vi "Teste234.vi"() -> ()   [LabVIEW 2019]
panel:
  out "tubo":i32(slide) scale=0.0..1950.0
  out "String lida em Caracter":string
  in  "home":bool
  in  "123":bool
  out "Altura Momentânea":i32
  in  "Parar":bool
  in  "Iniciar":bool
  in  "MWU2987":i16
  in  "MWU2986":i16
  in  "MWU2985":i16
  in  "MWU2984":i16
  in  "MWU2983":i16
  in  "MWU2982":i16
  in  "MWU2981":i16
  in  "MWU2980":i16
  in  "MWU2979":i16
  in  "MWU2978":i16
  in  "MWU2977":i16
  in  "MWU2976":i16
  in  "MWU2975":i16
  out "MWU1100":i16
  # "TESTE 234"
  # "mm"
  # "Teste destinado para verificar \no funcionamento mínimo do \nsistema\n Ao apertar em Iniciar, o sensor \nirá subir até 234mm e ficará \naguardando o usuário apertar o \nbotão HOME"
  # "Comando enviado"
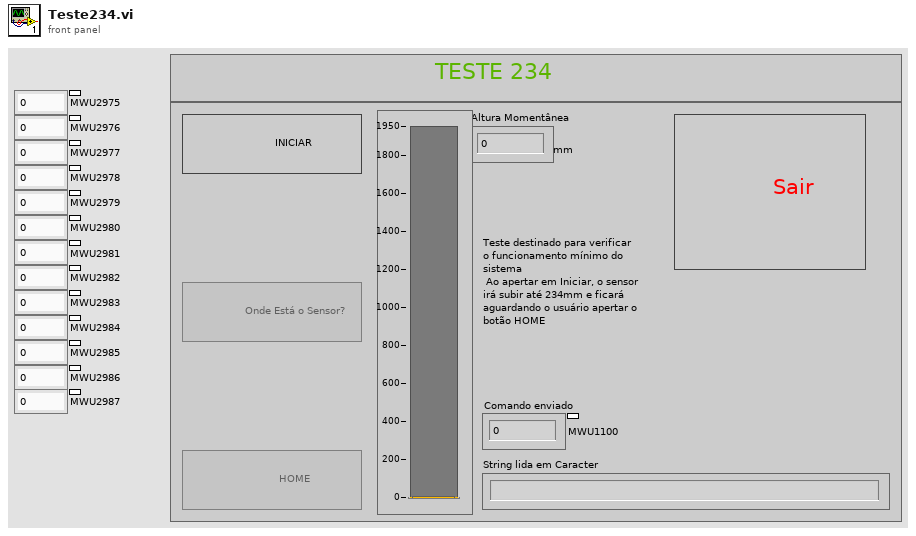
[diagram p1: front panel]
types:
  T1 = enum8{"Enabled", "Disabled", "Disabled and Grayed Out"}
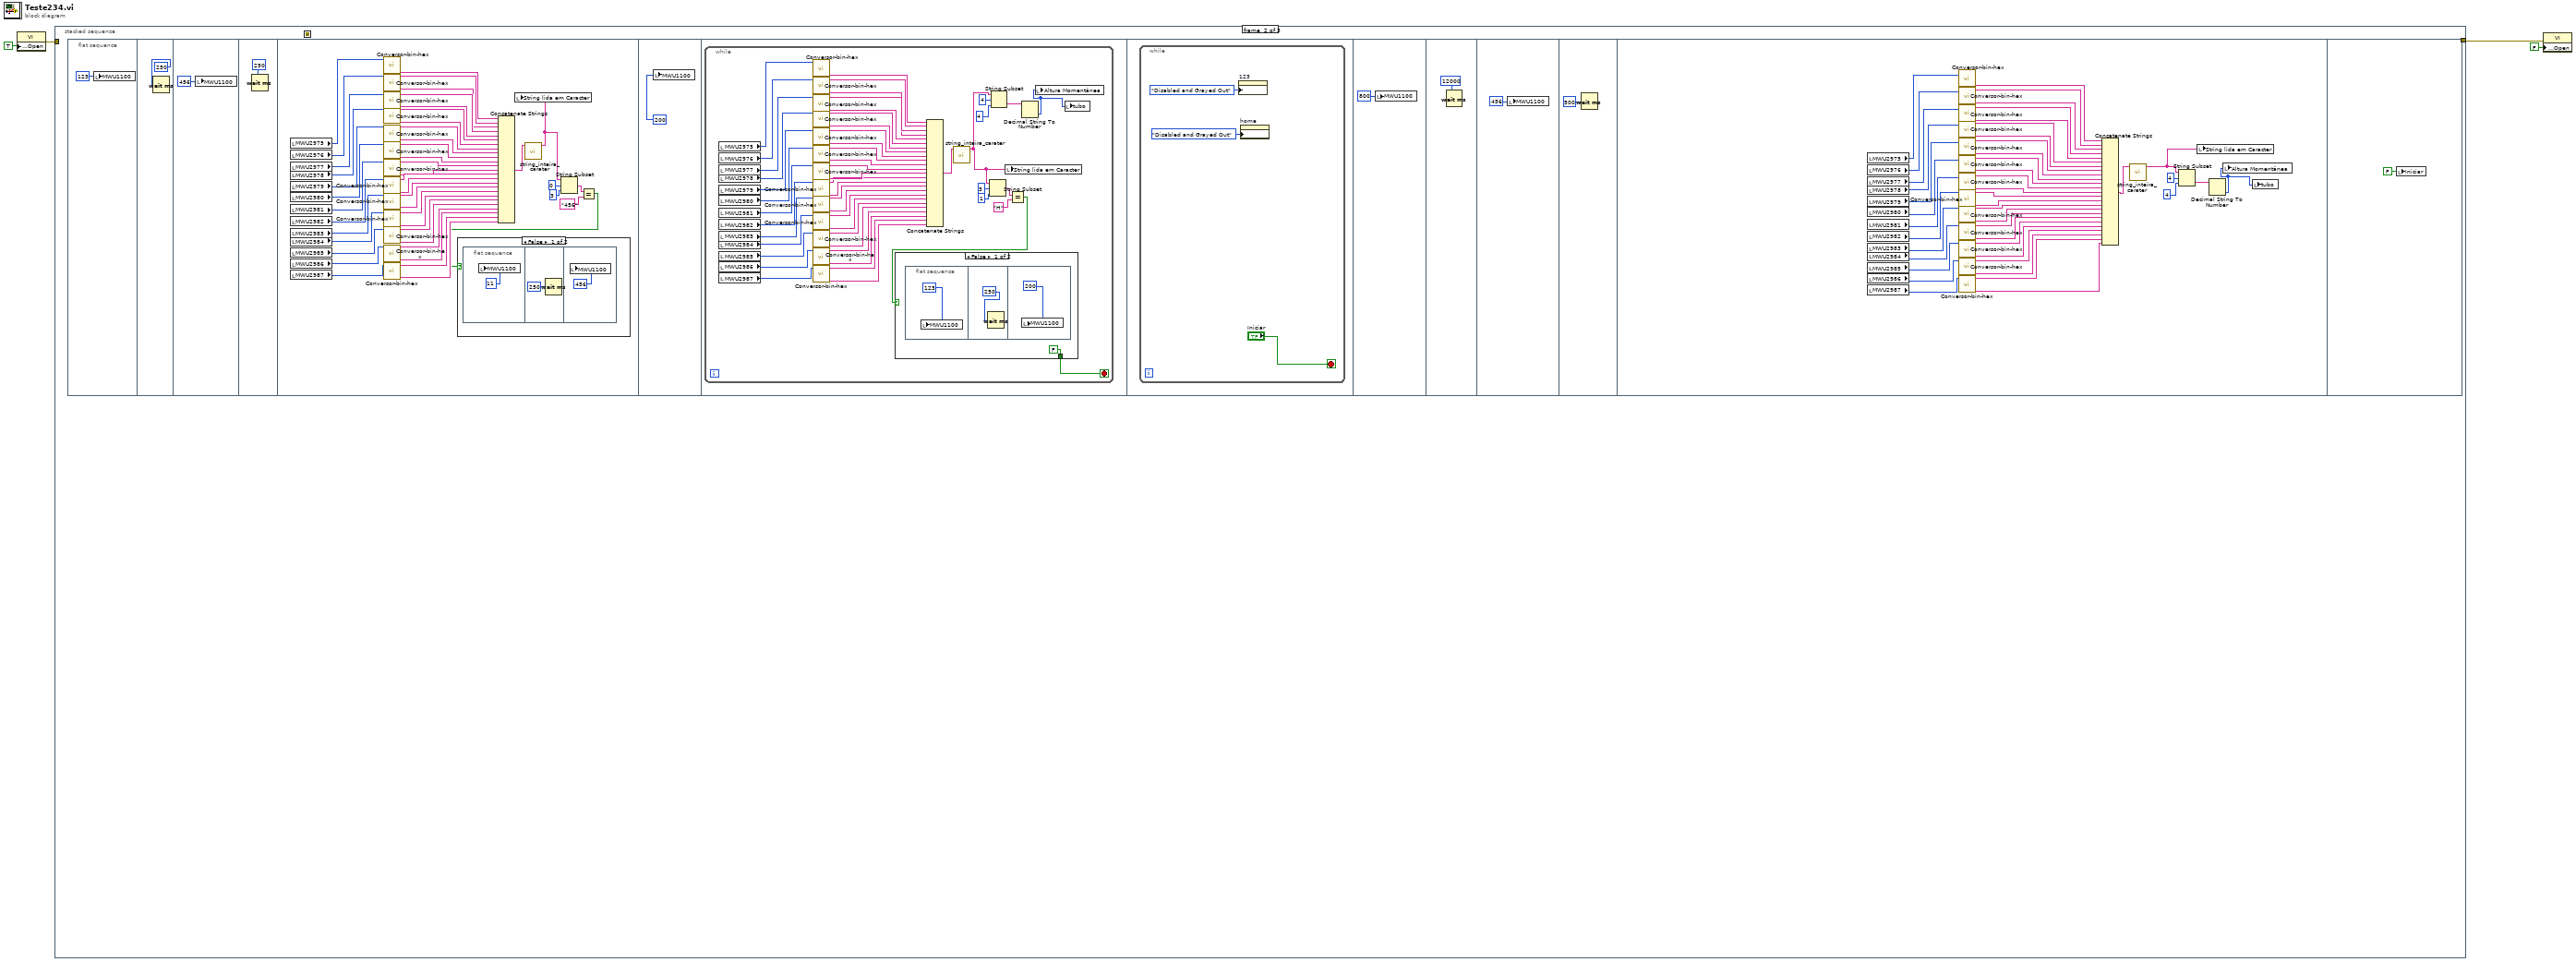
[diagram p0: block diagram]
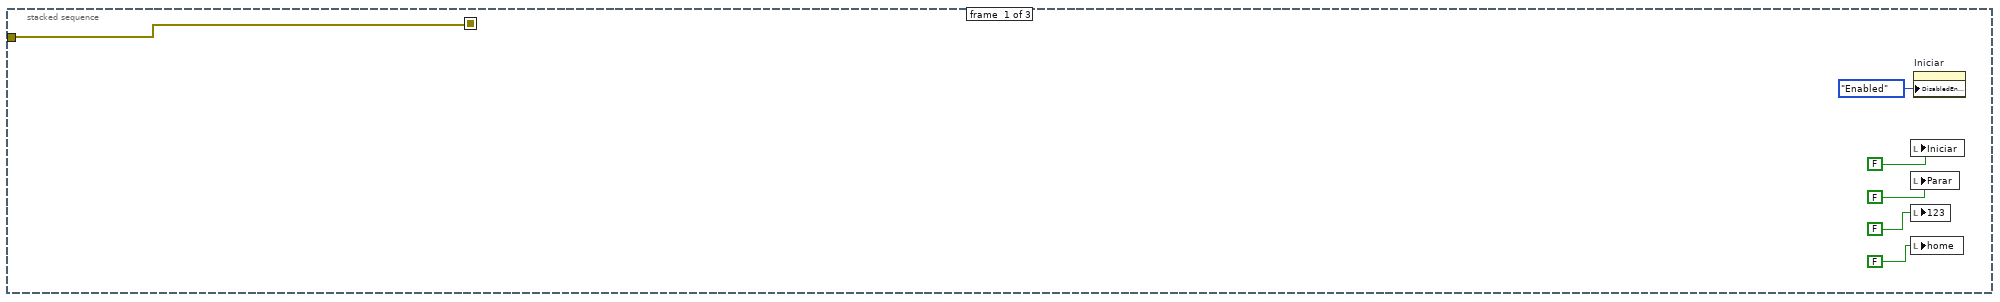
[diagram p2: hidden frame]
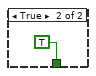
[diagram p4: hidden frame]
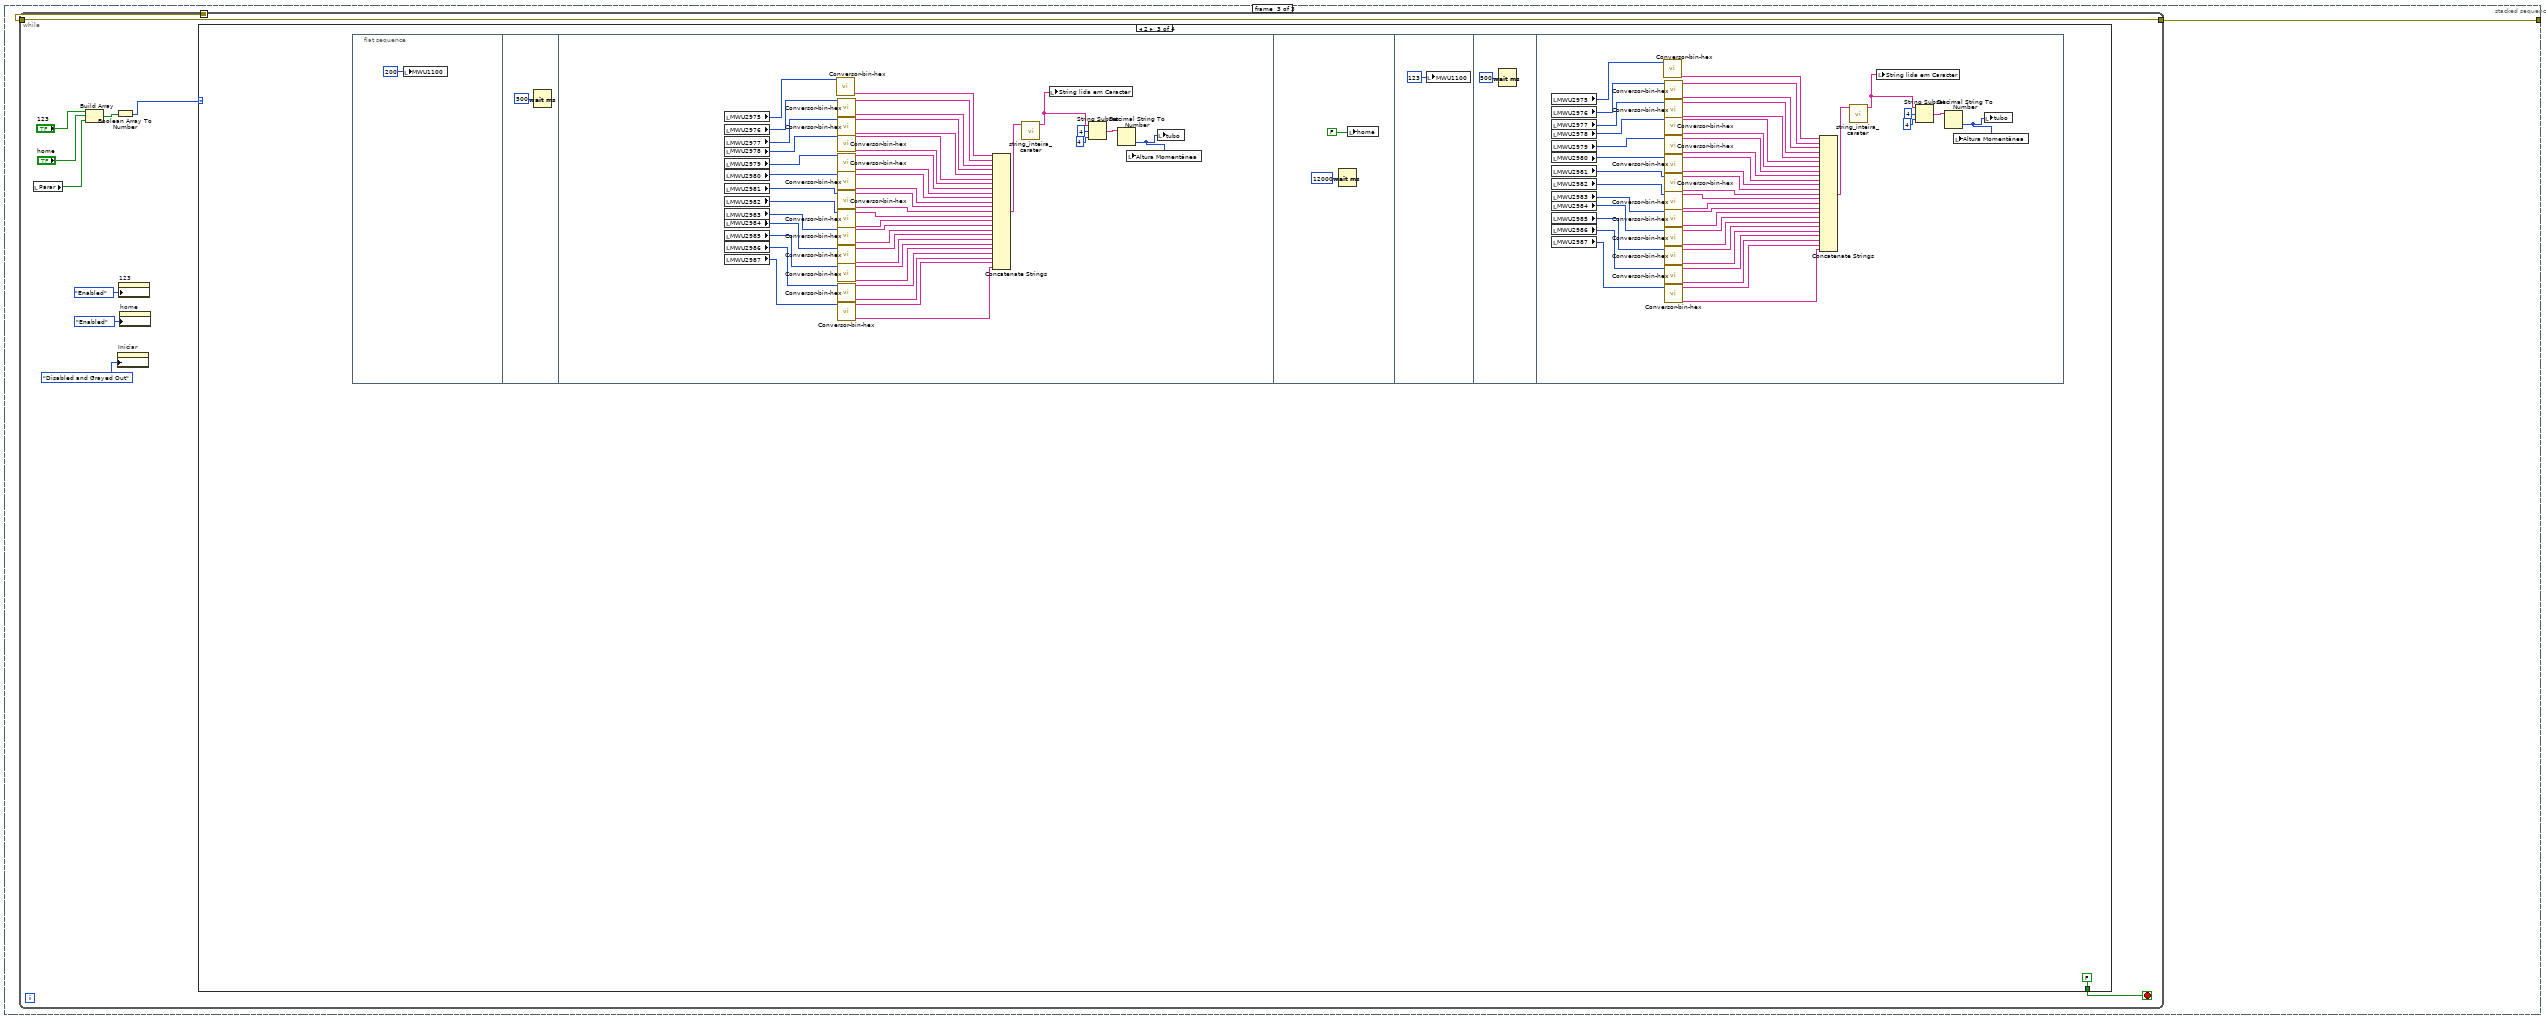
[diagram p5: hidden frame]
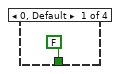
[diagram p6: hidden frame]
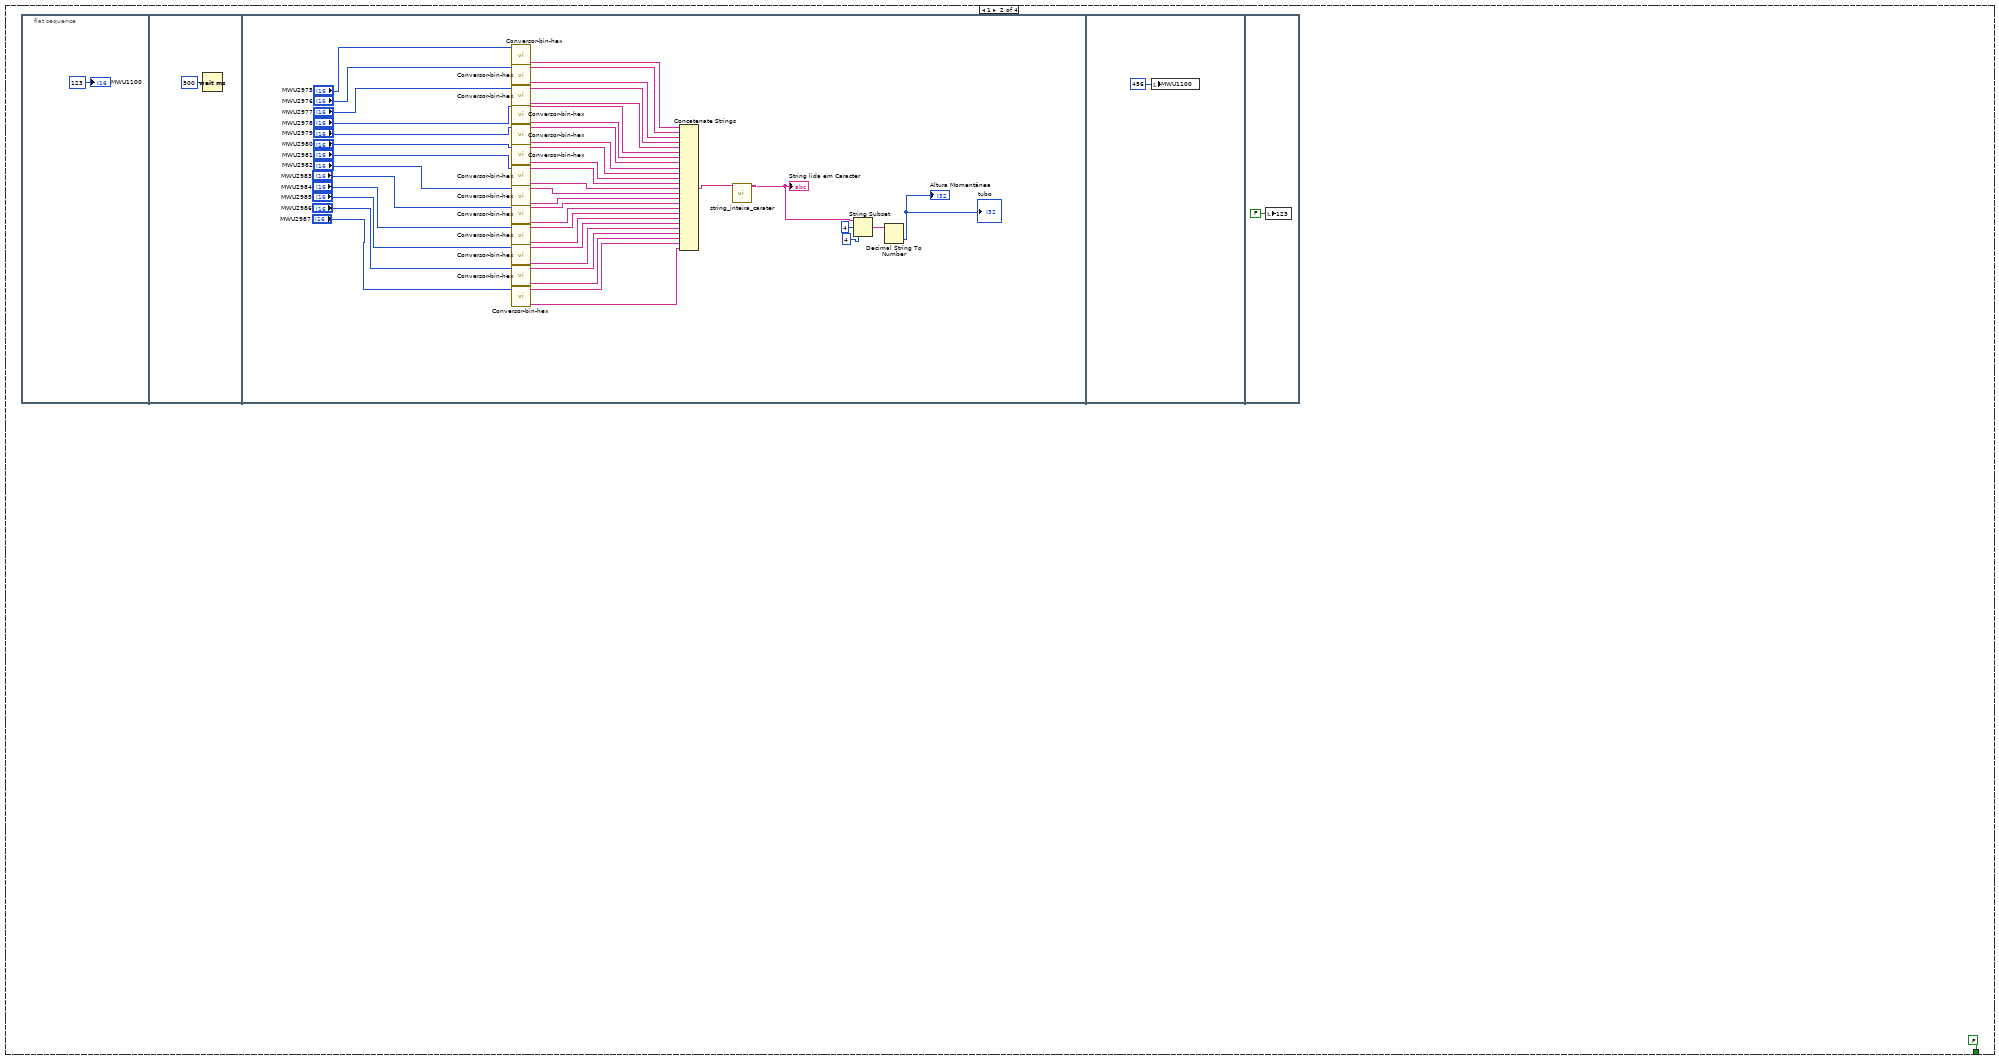
[diagram p7: hidden frame]
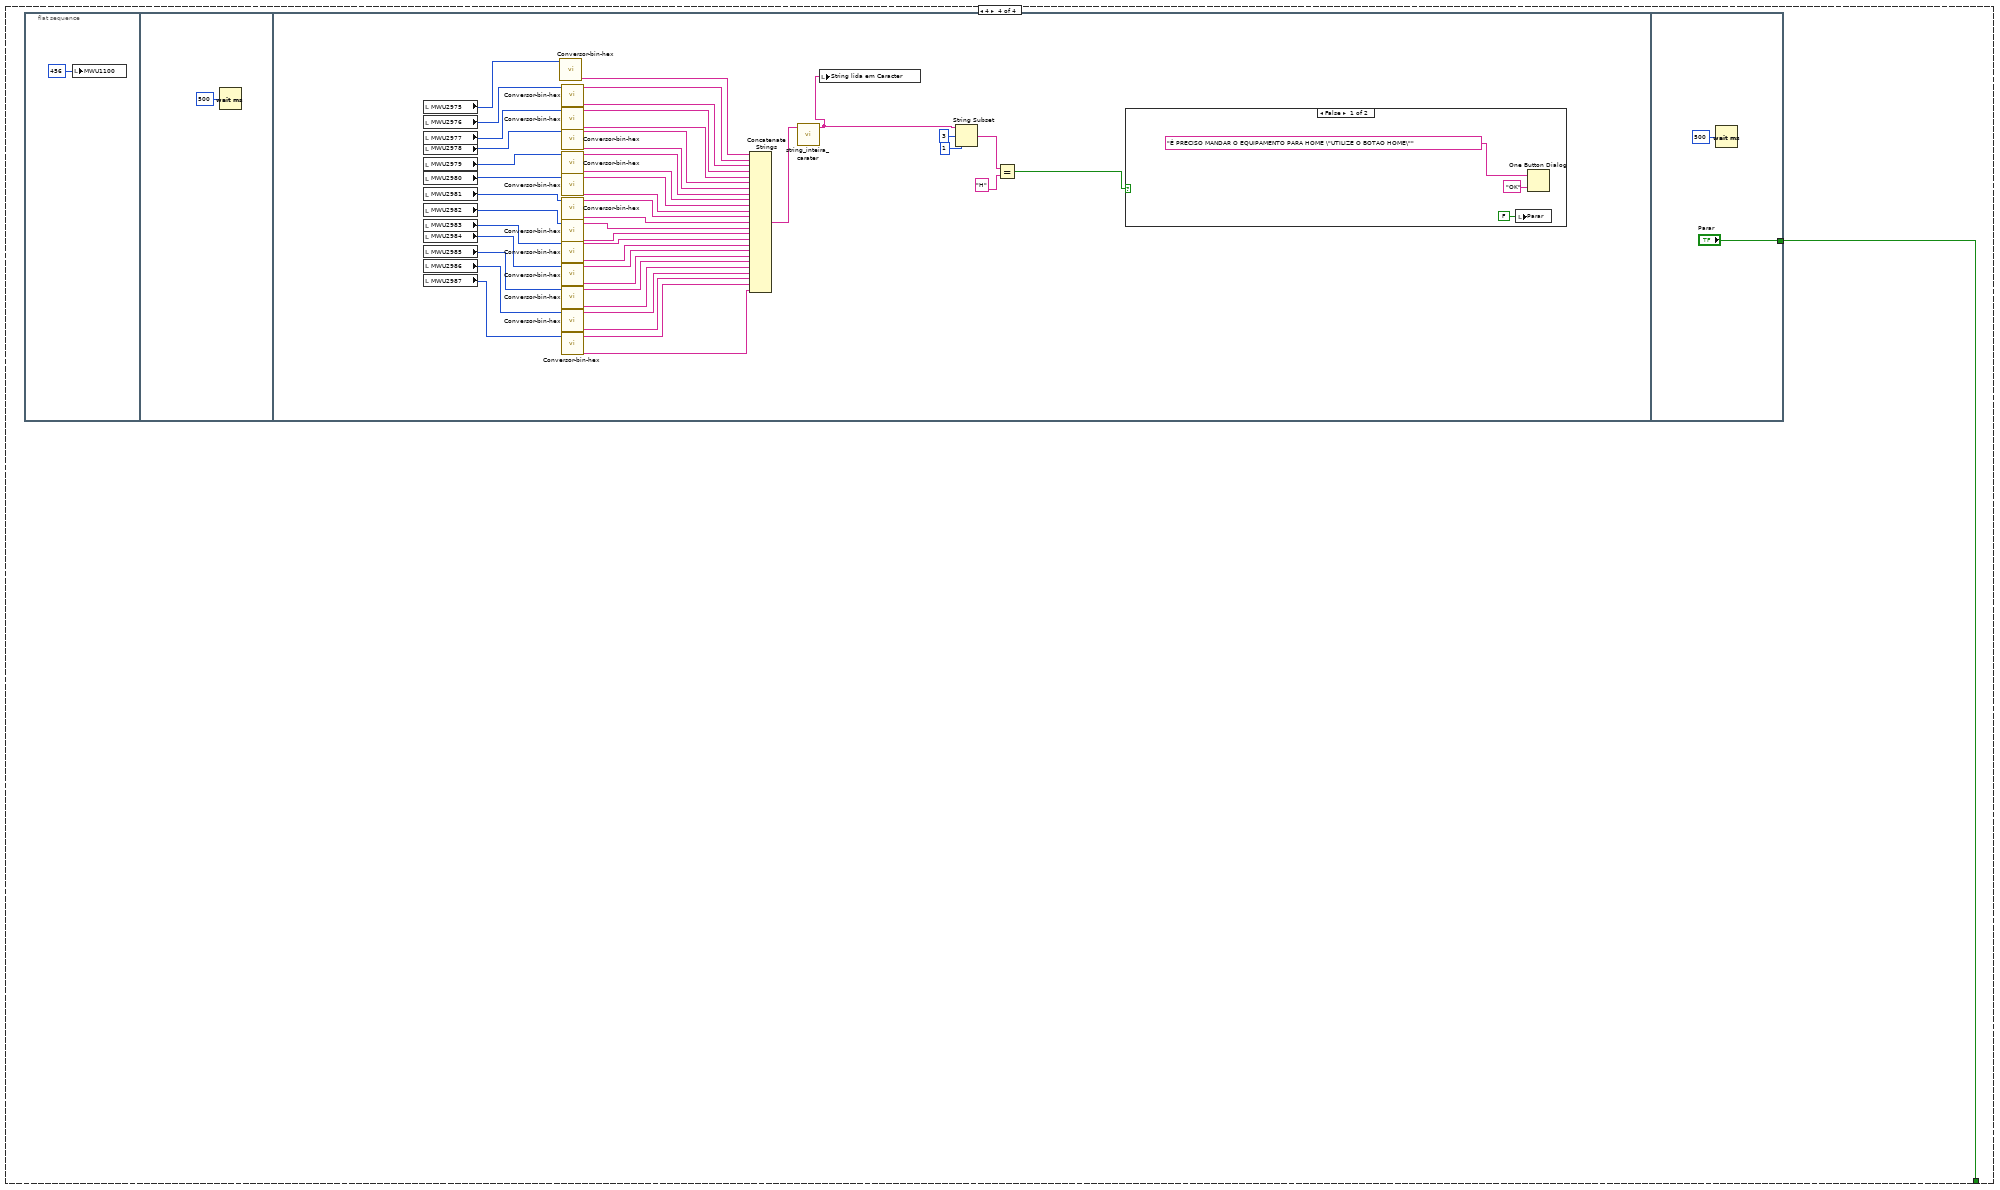
[diagram p8: hidden frame]
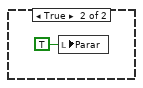
[diagram p9: hidden frame]
diagram:
  n1 = property class="VI"("Front Panel.Open"=TRUE ("Front Panel Window:Open")) -> (error out=w2:errorcluster)  [unwired: 2 in, 1 out]
  n2 = stacked-sequence {
    seq-local: [w10 _ _] -> [_ _ w172]
    tunnel: w2 -> [w10 _ _]
    tunnel: [_ _ w171] -> w1
    frame #0 {
      n3 = local write "Iniciar"(FALSE ("Iniciar")) -> ()
      n4 = local write "Parar"(FALSE ("Parar")) -> ()
      n5 = local write "123"(FALSE ("123")) -> ()
      n6 = local write "home"(FALSE ("home")) -> ()
      n7 = property on="Iniciar" class="Bool (strict)"("DisabledEnum"=T1."Enabled" ("Disabled")) -> ()  [unwired: 2 in, 2 out]
    }
    frame #1 {
      n8 = flat-sequence {
        frame #0 {
          n9 = local write "MWU1100"(i16 123 ("MWU1100")) -> ()
        }
        frame #1 {
          n10 = Wait (ms)(milliseconds to wait=u32 250) -> ()  [unwired: 1 out]
        }
        frame #2 {
          n11 = local write "MWU1100"(i16 456 ("MWU1100")) -> ()
        }
        frame #3 {
          n12 = Wait (ms)(milliseconds to wait=u32 250) -> ()  [unwired: 1 out]
        }
        frame #4 {
          n13 = local read "MWU2975"() -> (w33:i16)
          n14 = local read "MWU2976"() -> (w32:i16)
          n15 = local read "MWU2977"() -> (w31:i16)
          n16 = local read "MWU2978"() -> (w30:i16)
          n17 = local read "MWU2979"() -> (w29:i16)
          n18 = local read "MWU2980"() -> (w28:i16)
          n19 = local read "MWU2981"() -> (w27:i16)
          n20 = local read "MWU2982"() -> (w26:i16)
          n21 = local read "MWU2983"() -> (w25:i16)
          n22 = local read "MWU2984"() -> (w24:i16)
          n23 = local read "MWU2985"() -> (w23:i16)
          n24 = local read "MWU2986"() -> (w22:i16)
          n25 = local read "MWU2987"() -> (w21:i16)
          n26 = call "Conversor-bin-hex.vi"("Numeric"=w33) -> ("hex integer string"=w34:string)  [unwired: 9 in, 1 out]
          n27 = call "Conversor-bin-hex.vi"("Numeric"=w32) -> ("hex integer string"=w36:string, "hex integer string 2"=w35:string)  [unwired: 9 in]
          n28 = call "Conversor-bin-hex.vi"("Numeric"=w31) -> ("hex integer string"=w38:string, "hex integer string 2"=w37:string)  [unwired: 9 in]
          n29 = call "Conversor-bin-hex.vi"("Numeric"=w30) -> ("hex integer string"=w40:string, "hex integer string 2"=w39:string)  [unwired: 9 in]
          n30 = call "Conversor-bin-hex.vi"("Numeric"=w29) -> ("hex integer string"=w42:string, "hex integer string 2"=w41:string)  [unwired: 9 in]
          n31 = call "Conversor-bin-hex.vi"("Numeric"=w28) -> ("hex integer string"=w44:string, "hex integer string 2"=w43:string)  [unwired: 9 in]
          n32 = call "Conversor-bin-hex.vi"("Numeric"=w27) -> ("hex integer string"=w46:string, "hex integer string 2"=w45:string)  [unwired: 9 in]
          n33 = call "Conversor-bin-hex.vi"("Numeric"=w26) -> ("hex integer string"=w48:string, "hex integer string 2"=w47:string)  [unwired: 9 in]
          n34 = call "Conversor-bin-hex.vi"("Numeric"=w25) -> ("hex integer string"=w50:string, "hex integer string 2"=w49:string)  [unwired: 9 in]
          n35 = call "Conversor-bin-hex.vi"("Numeric"=w24) -> ("hex integer string"=w52:string, "hex integer string 2"=w51:string)  [unwired: 9 in]
          n36 = call "Conversor-bin-hex.vi"("Numeric"=w23) -> ("hex integer string"=w54:string, "hex integer string 2"=w53:string)  [unwired: 9 in]
          n37 = call "Conversor-bin-hex.vi"("Numeric"=w22) -> ("hex integer string"=w56:string, "hex integer string 2"=w55:string)  [unwired: 9 in]
          n38 = call "Conversor-bin-hex.vi"("Numeric"=w21) -> ("hex integer string"=w58:string, "hex integer string 2"=w57:string)  [unwired: 9 in]
          n39 = Concatenate Strings(w34, w35, w36, w37, w38, w39, w40, w41, w42, w43, w44, w45, w46, w47, w48, w49, w50, w51, w52, w53, w54, w55, w56, w57, w58) -> (w17:string)
          n40 = call "string_inteira_carater.vi"("String in"=w17) -> ("String out"=w16:string)  [unwired: 10 in]
          n41 = local write "String lida em Caracter"(w16) -> ()
          n42 = String Subset(string=w16, offset (0)=0, length (rest)=3 ("length (rest)")) -> (substring=w59:string)
          n43 = Equal?(x=w59, y="456") -> (x = y?=w15:bool)
          n44 = case shown="False" w15 {
            frame False {
              n45 = flat-sequence {
                frame #0 {
                  n46 = local write "MWU1100"(i16 11 ("MWU1100")) -> ()
                }
                frame #1 {
                  n47 = Wait (ms)(milliseconds to wait=u32 250) -> ()  [unwired: 1 out]
                }
                frame #2 {
                  n48 = local write "MWU1100"(i16 456 ("MWU1100")) -> ()
                }
              }
            }
            frame True {
            }
          }
        }
        frame #5 {
          n49 = local write "MWU1100"(i16 200 ("MWU1100")) -> ()
        }
        frame #6 {
          n50 = while {
            stop <- w70 stop-if-true
            n51 = local read "MWU2975"() -> (w97:i16)
            n52 = local read "MWU2976"() -> (w98:i16)
            n53 = local read "MWU2977"() -> (w99:i16)
            n54 = local read "MWU2978"() -> (w100:i16)
            n55 = local read "MWU2979"() -> (w101:i16)
            n56 = local read "MWU2980"() -> (w102:i16)
            n57 = local read "MWU2981"() -> (w103:i16)
            n58 = local read "MWU2982"() -> (w104:i16)
            n59 = local read "MWU2983"() -> (w105:i16)
            n60 = local read "MWU2984"() -> (w106:i16)
            n61 = local read "MWU2985"() -> (w107:i16)
            n62 = local read "MWU2986"() -> (w108:i16)
            n63 = local read "MWU2987"() -> (w109:i16)
            n64 = call "Conversor-bin-hex.vi"("Numeric"=w97) -> ("hex integer string"=w96:string)  [unwired: 9 in, 1 out]
            n65 = call "Conversor-bin-hex.vi"("Numeric"=w98) -> ("hex integer string"=w94:string, "hex integer string 2"=w95:string)  [unwired: 9 in]
            n66 = call "Conversor-bin-hex.vi"("Numeric"=w99) -> ("hex integer string"=w92:string, "hex integer string 2"=w93:string)  [unwired: 9 in]
            n67 = call "Conversor-bin-hex.vi"("Numeric"=w100) -> ("hex integer string"=w90:string, "hex integer string 2"=w91:string)  [unwired: 9 in]
            n68 = call "Conversor-bin-hex.vi"("Numeric"=w101) -> ("hex integer string"=w88:string, "hex integer string 2"=w89:string)  [unwired: 9 in]
            n69 = call "Conversor-bin-hex.vi"("Numeric"=w102) -> ("hex integer string"=w86:string, "hex integer string 2"=w87:string)  [unwired: 9 in]
            n70 = call "Conversor-bin-hex.vi"("Numeric"=w103) -> ("hex integer string"=w84:string, "hex integer string 2"=w85:string)  [unwired: 9 in]
            n71 = call "Conversor-bin-hex.vi"("Numeric"=w104) -> ("hex integer string"=w82:string, "hex integer string 2"=w83:string)  [unwired: 9 in]
            n72 = call "Conversor-bin-hex.vi"("Numeric"=w105) -> ("hex integer string"=w80:string, "hex integer string 2"=w81:string)  [unwired: 9 in]
            n73 = call "Conversor-bin-hex.vi"("Numeric"=w106) -> ("hex integer string"=w78:string, "hex integer string 2"=w79:string)  [unwired: 9 in]
            n74 = call "Conversor-bin-hex.vi"("Numeric"=w107) -> ("hex integer string"=w76:string, "hex integer string 2"=w77:string)  [unwired: 9 in]
            n75 = call "Conversor-bin-hex.vi"("Numeric"=w108) -> ("hex integer string"=w74:string, "hex integer string 2"=w75:string)  [unwired: 9 in]
            n76 = call "Conversor-bin-hex.vi"("Numeric"=w109) -> ("hex integer string"=w72:string, "hex integer string 2"=w73:string)  [unwired: 9 in]
            n77 = Concatenate Strings(w96, w95, w94, w93, w92, w91, w90, w89, w88, w87, w86, w85, w84, w83, w82, w81, w80, w79, w78, w77, w76, w75, w74, w73, w72) -> (w113:string)
            n78 = call "string_inteira_carater.vi"("String in"=w113) -> ("String out"=w65:string)  [unwired: 10 in]
            n79 = String Subset(string=w65, offset (0)=3, length (rest)=1 ("length (rest)")) -> (substring=w71:string)
            n80 = String Subset(string=w65, offset (0)=4, length (rest)=4 ("length (rest)")) -> (substring=w68:string)
            n81 = local write "String lida em Caracter"(w65) -> ()
            n82 = Equal?(x=w71, y="H") -> (x = y?=w64:bool)
            n83 = case shown="False" w64 {
              tunnel: [FALSE TRUE] -> w70
              frame False {
                n84 = flat-sequence {
                  frame #0 {
                    n85 = local write "MWU1100"(123) -> ()
                  }
                  frame #1 {
                    n86 = Wait (ms)(milliseconds to wait=250) -> ()  [unwired: 1 out]
                  }
                  frame #2 {
                    n87 = local write "MWU1100"(200) -> ()
                  }
                }
              }
              frame True {
              }
            }
            n88 = Decimal String To Number(string=w68) -> (number=w69:i32)  [unwired: 2 in, 1 out]
            n89 = local write "Altura Momentânea"(w69) -> ()
            n90 = local write "tubo"(w69) -> ()
          }
        }
        frame #7 {
          n91 = while {
            stop <- "Iniciar" stop-if-true
            n92 = property on="123" class="Bool (strict)"("DisabledEnum"=T1."Disabled and Grayed Out" ("Disabled")) -> ()  [unwired: 2 in, 2 out]
            n93 = property on="home" class="Bool (strict)"("DisabledEnum"=T1."Disabled and Grayed Out" ("Disabled")) -> ()  [unwired: 2 in, 2 out]
          }
        }
        frame #8 {
          n94 = local write "MWU1100"(i16 800 ("MWU1100")) -> ()
        }
        frame #9 {
          n95 = Wait (ms)(milliseconds to wait=u32 12000) -> ()  [unwired: 1 out]
        }
        frame #10 {
          n96 = local write "MWU1100"(i16 456 ("MWU1100")) -> ()
        }
        frame #11 {
          n97 = Wait (ms)(milliseconds to wait=u32 500) -> ()  [unwired: 1 out]
        }
        frame #12 {
          n98 = local read "MWU2975"() -> (w144:i16)
          n99 = local read "MWU2976"() -> (w143:i16)
          n100 = local read "MWU2977"() -> (w142:i16)
          n101 = local read "MWU2978"() -> (w141:i16)
          n102 = local read "MWU2979"() -> (w140:i16)
          n103 = local read "MWU2980"() -> (w139:i16)
          n104 = local read "MWU2981"() -> (w138:i16)
          n105 = local read "MWU2982"() -> (w137:i16)
          n106 = local read "MWU2983"() -> (w136:i16)
          n107 = local read "MWU2984"() -> (w135:i16)
          n108 = local read "MWU2985"() -> (w134:i16)
          n109 = local read "MWU2986"() -> (w133:i16)
          n110 = local read "MWU2987"() -> (w132:i16)
          n111 = call "Conversor-bin-hex.vi"("Numeric"=w144) -> ("hex integer string"=w145:string)  [unwired: 9 in, 1 out]
          n112 = call "Conversor-bin-hex.vi"("Numeric"=w143) -> ("hex integer string"=w147:string, "hex integer string 2"=w146:string)  [unwired: 9 in]
          n113 = call "Conversor-bin-hex.vi"("Numeric"=w142) -> ("hex integer string"=w149:string, "hex integer string 2"=w148:string)  [unwired: 9 in]
          n114 = call "Conversor-bin-hex.vi"("Numeric"=w141) -> ("hex integer string"=w151:string, "hex integer string 2"=w150:string)  [unwired: 9 in]
          n115 = call "Conversor-bin-hex.vi"("Numeric"=w140) -> ("hex integer string"=w153:string, "hex integer string 2"=w152:string)  [unwired: 9 in]
          n116 = call "Conversor-bin-hex.vi"("Numeric"=w139) -> ("hex integer string"=w155:string, "hex integer string 2"=w154:string)  [unwired: 9 in]
          n117 = call "Conversor-bin-hex.vi"("Numeric"=w138) -> ("hex integer string"=w157:string, "hex integer string 2"=w156:string)  [unwired: 9 in]
          n118 = call "Conversor-bin-hex.vi"("Numeric"=w137) -> ("hex integer string"=w159:string, "hex integer string 2"=w158:string)  [unwired: 9 in]
          n119 = call "Conversor-bin-hex.vi"("Numeric"=w136) -> ("hex integer string"=w161:string, "hex integer string 2"=w160:string)  [unwired: 9 in]
          n120 = call "Conversor-bin-hex.vi"("Numeric"=w135) -> ("hex integer string"=w163:string, "hex integer string 2"=w162:string)  [unwired: 9 in]
          n121 = call "Conversor-bin-hex.vi"("Numeric"=w134) -> ("hex integer string"=w165:string, "hex integer string 2"=w164:string)  [unwired: 9 in]
          n122 = call "Conversor-bin-hex.vi"("Numeric"=w133) -> ("hex integer string"=w167:string, "hex integer string 2"=w166:string)  [unwired: 9 in]
          n123 = call "Conversor-bin-hex.vi"("Numeric"=w132) -> ("hex integer string"=w169:string, "hex integer string 2"=w168:string)  [unwired: 9 in]
          n124 = Concatenate Strings(w145, w146, w147, w148, w149, w150, w151, w152, w153, w154, w155, w156, w157, w158, w159, w160, w161, w162, w163, w164, w165, w166, w167, w168, w169) -> (w131:string)
          n125 = call "string_inteira_carater.vi"("String in"=w131) -> ("String out"=w130:string)  [unwired: 10 in]
          n126 = String Subset(string=w130, offset (0)=4, length (rest)=4 ("length (rest)")) -> (substring=w127:string)
          n127 = local write "String lida em Caracter"(w130) -> ()
          n128 = Decimal String To Number(string=w127) -> (number=w126:i32)  [unwired: 2 in, 1 out]
          n129 = local write "Altura Momentânea"(w126) -> ()
          n130 = local write "tubo"(w126) -> ()
        }
        frame #13 {
          n131 = local write "Iniciar"(FALSE ("Iniciar")) -> ()
        }
      }
    }
    frame #2 {
      n132 = while {
        tunnel: w172 -> [w182]
        tunnel: [w182] -> w171
        stop <- w176 stop-if-true
        n133 = local read "Parar"() -> (w177:bool)
        n134 = Build Array("123", "home", w177) -> (w179:bool[])
        n135 = Boolean Array To Number(Boolean array=w179) -> (number=w178:u32)
        n136 = property on="Iniciar" class="Bool (strict)"("DisabledEnum"=T1."Disabled and Grayed Out" ("Disabled")) -> ()  [unwired: 2 in, 2 out]
        n137 = property on="123" class="Bool (strict)"("DisabledEnum"=T1."Enabled" ("Disabled")) -> ()  [unwired: 2 in, 2 out]
        n138 = property on="home" class="Bool (strict)"("DisabledEnum"=T1."Enabled" ("Disabled")) -> ()  [unwired: 2 in, 2 out]
        n139 = case shown="2" w178 {
          tunnel: [FALSE ("Parar") FALSE ("Parar") FALSE ("Parar") w328] -> w176
          frame 0, Default {
          }
          frame 1 {
            n140 = flat-sequence {
              frame #0 {
                "MWU1100" <- i16 123 ("MWU1100")
              }
              frame #1 {
                n141 = Wait (ms)(milliseconds to wait=u32 500) -> ()  [unwired: 1 out]
              }
              frame #2 {
                n142 = call "Conversor-bin-hex.vi"("Numeric"="MWU2975") -> ("hex integer string"=w230:string)  [unwired: 9 in, 1 out]
                n143 = call "Conversor-bin-hex.vi"("Numeric"="MWU2976") -> ("hex integer string"=w228:string, "hex integer string 2"=w229:string)  [unwired: 9 in]
                n144 = call "Conversor-bin-hex.vi"("Numeric"="MWU2977") -> ("hex integer string"=w226:string, "hex integer string 2"=w227:string)  [unwired: 9 in]
                n145 = call "Conversor-bin-hex.vi"("Numeric"="MWU2978") -> ("hex integer string"=w224:string, "hex integer string 2"=w225:string)  [unwired: 9 in]
                n146 = call "Conversor-bin-hex.vi"("Numeric"="MWU2979") -> ("hex integer string"=w222:string, "hex integer string 2"=w223:string)  [unwired: 9 in]
                n147 = call "Conversor-bin-hex.vi"("Numeric"="MWU2980") -> ("hex integer string"=w220:string, "hex integer string 2"=w221:string)  [unwired: 9 in]
                n148 = call "Conversor-bin-hex.vi"("Numeric"="MWU2981") -> ("hex integer string"=w218:string, "hex integer string 2"=w219:string)  [unwired: 9 in]
                n149 = call "Conversor-bin-hex.vi"("Numeric"="MWU2982") -> ("hex integer string"=w216:string, "hex integer string 2"=w217:string)  [unwired: 9 in]
                n150 = call "Conversor-bin-hex.vi"("Numeric"="MWU2983") -> ("hex integer string"=w214:string, "hex integer string 2"=w215:string)  [unwired: 9 in]
                n151 = call "Conversor-bin-hex.vi"("Numeric"="MWU2984") -> ("hex integer string"=w212:string, "hex integer string 2"=w213:string)  [unwired: 9 in]
                n152 = call "Conversor-bin-hex.vi"("Numeric"="MWU2985") -> ("hex integer string"=w210:string, "hex integer string 2"=w211:string)  [unwired: 9 in]
                n153 = call "Conversor-bin-hex.vi"("Numeric"="MWU2986") -> ("hex integer string"=w208:string, "hex integer string 2"=w209:string)  [unwired: 9 in]
                n154 = call "Conversor-bin-hex.vi"("Numeric"="MWU2987") -> ("hex integer string"=w206:string, "hex integer string 2"=w207:string)  [unwired: 9 in]
                n155 = Concatenate Strings(w230, w229, w228, w227, w226, w225, w224, w223, w222, w221, w220, w219, w218, w217, w216, w215, w214, w213, w212, w211, w210, w209, w208, w207, w206) -> (w192:string)
                n156 = call "string_inteira_carater.vi"("String in"=w192) -> ("String out"=w190:string)  [unwired: 10 in]
                "String lida em Caracter" <- w190
                n157 = String Subset(string=w190, offset (0)=4, length (rest)=4 ("length (rest)")) -> (substring=w188:string)
                n158 = Decimal String To Number(string=w188) -> (number=→"Altura Momentânea" →"tubo":i32)  [unwired: 2 in, 1 out]
              }
              frame #3 {
                n159 = local write "MWU1100"(i16 456 ("MWU1100")) -> ()
              }
              frame #4 {
                n160 = local write "123"(FALSE ("123")) -> ()
              }
            }
          }
          frame 2 {
            n161 = flat-sequence {
              frame #0 {
                n162 = local write "MWU1100"(i16 200 ("MWU1100")) -> ()
              }
              frame #1 {
                n163 = Wait (ms)(milliseconds to wait=u32 500) -> ()  [unwired: 1 out]
              }
              frame #2 {
                n164 = local read "MWU2975"() -> (w255:i16)
                n165 = local read "MWU2976"() -> (w254:i16)
                n166 = local read "MWU2977"() -> (w253:i16)
                n167 = local read "MWU2978"() -> (w252:i16)
                n168 = local read "MWU2979"() -> (w251:i16)
                n169 = local read "MWU2980"() -> (w250:i16)
                n170 = local read "MWU2981"() -> (w249:i16)
                n171 = local read "MWU2982"() -> (w248:i16)
                n172 = local read "MWU2983"() -> (w247:i16)
                n173 = local read "MWU2984"() -> (w246:i16)
                n174 = local read "MWU2985"() -> (w245:i16)
                n175 = local read "MWU2986"() -> (w244:i16)
                n176 = local read "MWU2987"() -> (w243:i16)
                n177 = call "Conversor-bin-hex.vi"("Numeric"=w255) -> ("hex integer string"=w279:string)  [unwired: 9 in, 1 out]
                n178 = call "Conversor-bin-hex.vi"("Numeric"=w254) -> ("hex integer string"=w277:string, "hex integer string 2"=w278:string)  [unwired: 9 in]
                n179 = call "Conversor-bin-hex.vi"("Numeric"=w253) -> ("hex integer string"=w275:string, "hex integer string 2"=w276:string)  [unwired: 9 in]
                n180 = call "Conversor-bin-hex.vi"("Numeric"=w252) -> ("hex integer string"=w273:string, "hex integer string 2"=w274:string)  [unwired: 9 in]
                n181 = call "Conversor-bin-hex.vi"("Numeric"=w251) -> ("hex integer string"=w271:string, "hex integer string 2"=w272:string)  [unwired: 9 in]
                n182 = call "Conversor-bin-hex.vi"("Numeric"=w250) -> ("hex integer string"=w269:string, "hex integer string 2"=w270:string)  [unwired: 9 in]
                n183 = call "Conversor-bin-hex.vi"("Numeric"=w249) -> ("hex integer string"=w267:string, "hex integer string 2"=w268:string)  [unwired: 9 in]
                n184 = call "Conversor-bin-hex.vi"("Numeric"=w248) -> ("hex integer string"=w265:string, "hex integer string 2"=w266:string)  [unwired: 9 in]
                n185 = call "Conversor-bin-hex.vi"("Numeric"=w247) -> ("hex integer string"=w263:string, "hex integer string 2"=w264:string)  [unwired: 9 in]
                n186 = call "Conversor-bin-hex.vi"("Numeric"=w246) -> ("hex integer string"=w261:string, "hex integer string 2"=w262:string)  [unwired: 9 in]
                n187 = call "Conversor-bin-hex.vi"("Numeric"=w245) -> ("hex integer string"=w259:string, "hex integer string 2"=w260:string)  [unwired: 9 in]
                n188 = call "Conversor-bin-hex.vi"("Numeric"=w244) -> ("hex integer string"=w257:string, "hex integer string 2"=w258:string)  [unwired: 9 in]
                n189 = call "Conversor-bin-hex.vi"("Numeric"=w243) -> ("hex integer string"=w242:string, "hex integer string 2"=w256:string)  [unwired: 9 in]
                n190 = Concatenate Strings(w279, w278, w277, w276, w275, w274, w273, w272, w271, w270, w269, w268, w267, w266, w265, w264, w263, w262, w261, w260, w259, w258, w257, w256, w242) -> (w241:string)
                n191 = call "string_inteira_carater.vi"("String in"=w241) -> ("String out"=w237:string)  [unwired: 10 in]
                n192 = local write "String lida em Caracter"(w237) -> ()
                n193 = String Subset(string=w237, offset (0)=4, length (rest)=4 ("length (rest)")) -> (substring=w240:string)
                n194 = Decimal String To Number(string=w240) -> (number=w236:i32)  [unwired: 2 in, 1 out]
                n195 = local write "Altura Momentânea"(w236) -> ()
                n196 = local write "tubo"(w236) -> ()
              }
              frame #3 {
                n197 = Wait (ms)(milliseconds to wait=u32 12000) -> ()  [unwired: 1 out]
                n198 = local write "home"(FALSE ("200")) -> ()
              }
              frame #4 {
                n199 = local write "MWU1100"(i16 123 ("MWU1100")) -> ()
              }
              frame #5 {
                n200 = Wait (ms)(milliseconds to wait=u32 500) -> ()  [unwired: 1 out]
              }
              frame #6 {
                n201 = local read "MWU2975"() -> (w308:i16)
                n202 = local read "MWU2976"() -> (w309:i16)
                n203 = local read "MWU2977"() -> (w310:i16)
                n204 = local read "MWU2978"() -> (w311:i16)
                n205 = local read "MWU2979"() -> (w312:i16)
                n206 = local read "MWU2980"() -> (w313:i16)
                n207 = local read "MWU2981"() -> (w314:i16)
                n208 = local read "MWU2982"() -> (w315:i16)
                n209 = local read "MWU2983"() -> (w316:i16)
                n210 = local read "MWU2984"() -> (w317:i16)
                n211 = local read "MWU2985"() -> (w318:i16)
                n212 = local read "MWU2986"() -> (w319:i16)
                n213 = local read "MWU2987"() -> (w320:i16)
                n214 = call "Conversor-bin-hex.vi"("Numeric"=w308) -> ("hex integer string"=w284:string)  [unwired: 9 in, 1 out]
                n215 = call "Conversor-bin-hex.vi"("Numeric"=w309) -> ("hex integer string"=w286:string, "hex integer string 2"=w285:string)  [unwired: 9 in]
                n216 = call "Conversor-bin-hex.vi"("Numeric"=w310) -> ("hex integer string"=w288:string, "hex integer string 2"=w287:string)  [unwired: 9 in]
                n217 = call "Conversor-bin-hex.vi"("Numeric"=w311) -> ("hex integer string"=w290:string, "hex integer string 2"=w289:string)  [unwired: 9 in]
                n218 = call "Conversor-bin-hex.vi"("Numeric"=w312) -> ("hex integer string"=w292:string, "hex integer string 2"=w291:string)  [unwired: 9 in]
                n219 = call "Conversor-bin-hex.vi"("Numeric"=w313) -> ("hex integer string"=w294:string, "hex integer string 2"=w293:string)  [unwired: 9 in]
                n220 = call "Conversor-bin-hex.vi"("Numeric"=w314) -> ("hex integer string"=w296:string, "hex integer string 2"=w295:string)  [unwired: 9 in]
                n221 = call "Conversor-bin-hex.vi"("Numeric"=w315) -> ("hex integer string"=w298:string, "hex integer string 2"=w297:string)  [unwired: 9 in]
                n222 = call "Conversor-bin-hex.vi"("Numeric"=w316) -> ("hex integer string"=w300:string, "hex integer string 2"=w299:string)  [unwired: 9 in]
                n223 = call "Conversor-bin-hex.vi"("Numeric"=w317) -> ("hex integer string"=w302:string, "hex integer string 2"=w301:string)  [unwired: 9 in]
                n224 = call "Conversor-bin-hex.vi"("Numeric"=w318) -> ("hex integer string"=w304:string, "hex integer string 2"=w303:string)  [unwired: 9 in]
                n225 = call "Conversor-bin-hex.vi"("Numeric"=w319) -> ("hex integer string"=w306:string, "hex integer string 2"=w305:string)  [unwired: 9 in]
                n226 = call "Conversor-bin-hex.vi"("Numeric"=w320) -> ("hex integer string"=w321:string, "hex integer string 2"=w307:string)  [unwired: 9 in]
                n227 = Concatenate Strings(w284, w285, w286, w287, w288, w289, w290, w291, w292, w293, w294, w295, w296, w297, w298, w299, w300, w301, w302, w303, w304, w305, w306, w307, w321) -> (w322:string)
                n228 = call "string_inteira_carater.vi"("String in"=w322) -> ("String out"=w326:string)  [unwired: 10 in]
                n229 = local write "String lida em Caracter"(w326) -> ()
                n230 = String Subset(string=w326, offset (0)=4, length (rest)=4 ("length (rest)")) -> (substring=w323:string)
                n231 = Decimal String To Number(string=w323) -> (number=w327:i32)  [unwired: 2 in, 1 out]
                n232 = local write "Altura Momentânea"(w327) -> ()
                n233 = local write "tubo"(w327) -> ()
              }
            }
          }
          frame 4 {
            n234 = flat-sequence {
              tunnel: ["Parar"] -> w328
              frame #0 {
                n235 = local write "MWU1100"(i16 456 ("MWU1100")) -> ()
              }
              frame #1 {
                n236 = Wait (ms)(milliseconds to wait=u32 500) -> ()  [unwired: 1 out]
              }
              frame #2 {
                n237 = local read "MWU2975"() -> (w351:i16)
                n238 = local read "MWU2976"() -> (w350:i16)
                n239 = local read "MWU2977"() -> (w349:i16)
                n240 = local read "MWU2978"() -> (w348:i16)
                n241 = local read "MWU2979"() -> (w347:i16)
                n242 = local read "MWU2980"() -> (w346:i16)
                n243 = local read "MWU2981"() -> (w345:i16)
                n244 = local read "MWU2982"() -> (w344:i16)
                n245 = local read "MWU2983"() -> (w343:i16)
                n246 = local read "MWU2984"() -> (w342:i16)
                n247 = local read "MWU2985"() -> (w341:i16)
                n248 = local read "MWU2986"() -> (w340:i16)
                n249 = local read "MWU2987"() -> (w339:i16)
                n250 = call "Conversor-bin-hex.vi"("Numeric"=w351) -> ("hex integer string"=w375:string)  [unwired: 9 in, 1 out]
                n251 = call "Conversor-bin-hex.vi"("Numeric"=w350) -> ("hex integer string"=w373:string, "hex integer string 2"=w374:string)  [unwired: 9 in]
                n252 = call "Conversor-bin-hex.vi"("Numeric"=w349) -> ("hex integer string"=w371:string, "hex integer string 2"=w372:string)  [unwired: 9 in]
                n253 = call "Conversor-bin-hex.vi"("Numeric"=w348) -> ("hex integer string"=w369:string, "hex integer string 2"=w370:string)  [unwired: 9 in]
                n254 = call "Conversor-bin-hex.vi"("Numeric"=w347) -> ("hex integer string"=w367:string, "hex integer string 2"=w368:string)  [unwired: 9 in]
                n255 = call "Conversor-bin-hex.vi"("Numeric"=w346) -> ("hex integer string"=w365:string, "hex integer string 2"=w366:string)  [unwired: 9 in]
                n256 = call "Conversor-bin-hex.vi"("Numeric"=w345) -> ("hex integer string"=w363:string, "hex integer string 2"=w364:string)  [unwired: 9 in]
                n257 = call "Conversor-bin-hex.vi"("Numeric"=w344) -> ("hex integer string"=w361:string, "hex integer string 2"=w362:string)  [unwired: 9 in]
                n258 = call "Conversor-bin-hex.vi"("Numeric"=w343) -> ("hex integer string"=w359:string, "hex integer string 2"=w360:string)  [unwired: 9 in]
                n259 = call "Conversor-bin-hex.vi"("Numeric"=w342) -> ("hex integer string"=w357:string, "hex integer string 2"=w358:string)  [unwired: 9 in]
                n260 = call "Conversor-bin-hex.vi"("Numeric"=w341) -> ("hex integer string"=w355:string, "hex integer string 2"=w356:string)  [unwired: 9 in]
                n261 = call "Conversor-bin-hex.vi"("Numeric"=w340) -> ("hex integer string"=w353:string, "hex integer string 2"=w354:string)  [unwired: 9 in]
                n262 = call "Conversor-bin-hex.vi"("Numeric"=w339) -> ("hex integer string"=w335:string, "hex integer string 2"=w352:string)  [unwired: 9 in]
                n263 = Concatenate Strings(w375, w374, w373, w372, w371, w370, w369, w368, w367, w366, w365, w364, w363, w362, w361, w360, w359, w358, w357, w356, w355, w354, w353, w352, w335) -> (w332:string)
                n264 = call "string_inteira_carater.vi"("String in"=w332) -> ("String out"=w331:string)  [unwired: 10 in]
                n265 = local write "String lida em Caracter"(w331) -> ()
                n266 = String Subset(string=w331, offset (0)=3, length (rest)=1 ("length (rest)")) -> (substring=w333:string)
                n267 = Equal?(x=w333, y="H") -> (x = y?=w334:bool)
                n268 = case shown="False" w334 {
                  frame False {
                    n269 = local write "Parar"(FALSE ("Parar")) -> ()
                    n270 = One Button Dialog(message="É PRECISO MANDAR O EQUIPAMENTO PARA HOME \"UTILIZE O BOTAO HOME\"", button name ("OK")="OK") -> ()  [unwired: 1 out]
                  }
                  frame True {
                    n271 = local write "Parar"(TRUE ("Parar")) -> ()
                  }
                }
              }
              frame #3 {
                n272 = Wait (ms)(milliseconds to wait=u32 500) -> ()  [unwired: 1 out]
              }
            }
          }
        }
      }
    }
  }
  n273 = property class="VI"(error in=w1, "Front Panel.Open"=FALSE ("Front Panel Window:Open")) -> ()  [unwired: 1 in, 2 out]
